vi "Robot Global Data.vi"() -> ()   [LabVIEW 2017]
doc: "This global VI can contain as many global variables as you need. Place a control on the panel, give it a good name. To read or write to it from a VI, drag the icon to the diagram of that VI. You can also drag from the project. Click on the node to change which global you access. You shouldn't have multiple locations writing to a global or it will cause a race-condition."
uses:
  <vilib>/Rock Robotics/WPI/Camera/WPI_CameraImageSize.ctl
  <vilib>/Rock Robotics/WPI/DriverStation/WPI_DriverStationRobotMode2.ctl
  Common Code/Dashboard Control Data.ctl
  Common Code/Drivetrain Command Cluster.ctl
  Common Code/Drivetrain Mode.ctl
  Common Code/Drivetrain Status Cluster.ctl
  Common Code/Climb Command Cluster.ctl
  Common Code/Climb Status Cluster.ctl
  Common Code/DT Encoder Values.ctl
panel:
  in  "Drivetrain Encoder Values":T1
  in  "Climb Status Cluster":T2
  in  "Climb Command Cluster":T3
  out "Drivetrain Status Cluster":T4 {"Gyro" scale=-180.0..180.0}
  in  "Drivetrain Command Cluster":T6
  in  "Dashboard Control Data":T7
  in  "Driver Station IP":dbl
  in  "Robot Mode":T8
  in  "image size":T9=enum."320x240"
  in  "Enable Vision":bool
  # "Dashboard"
  # "Drivetrain"
  # "Intake"
  # "Climber"
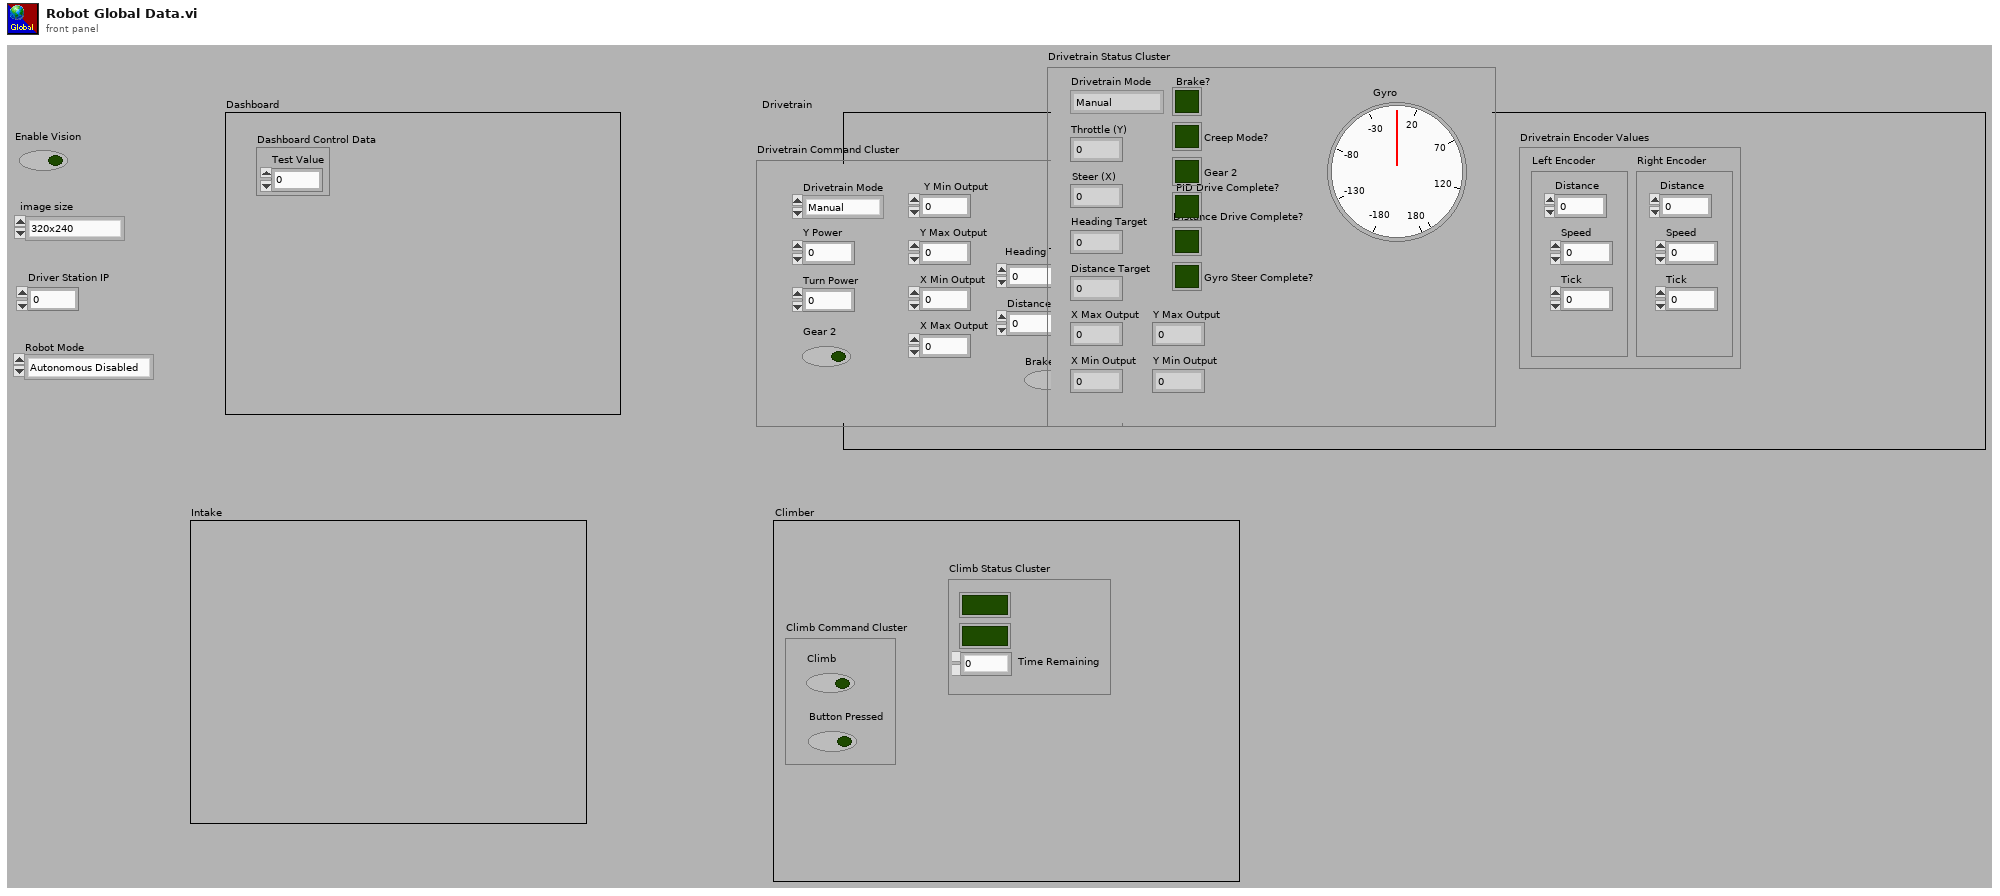
[diagram p1: front panel]
types:
  T1 = typedef "DT Encoder Values.ctl" = cluster{"Left Encoder":cluster{"Distance":dbl, "Speed":dbl, "Tick":dbl}, "Right Encoder":cluster{"Distance":dbl, "Speed":dbl, "Tick":dbl}}
  T2 = typedef "Climb Status Cluster.ctl" = cluster{"Climb":bool, "Button Pressed":bool, "Time Remaining":dbl}
  T3 = typedef "Climb Command Cluster.ctl" = cluster{"Climb":bool, "Button Pressed":bool}
  T4 = typedef "Drivetrain Status Cluster.ctl" = cluster{"Throttle (Y)":dbl, "Steer (X)":dbl, "Drivetrain Mode":T5, "Brake?":bool, "Distance Drive Complete?":bool, "PID Drive Complete?":bool, "Creep Mode?":bool, "Gyro Steer Complete?":bool, "Gyro":dbl, "X Max Output":dbl, "X Min Output":dbl, "Y Max Output ":dbl, "Y Min Output":dbl, "Heading Target":dbl, "Distance Target":dbl, "Gear 2":bool}
  T5 = typedef "Drivetrain Mode.ctl" = enum16{"Manual", "Gyro Steer", "PID Drive", "Distance Drive", "Autonomous"}
  T6 = typedef "Drivetrain Command Cluster.ctl" = cluster{"Y Power":dbl, "Turn Power":dbl, "Drivetrain Mode":T5, "Gear 2":bool, "Y Min Output":dbl, "Y Max Output":dbl, "X Min Output":dbl, "X Max Output":dbl, "Heading Target":dbl, "Distance Target":dbl, "Brake?":bool}
  T7 = typedef "Dashboard Control Data.ctl" = cluster{"Test Value":dbl}
  T8 = typedef "WPI_DriverStationRobotMode2.ctl" = enum16{"Autonomous Disabled", "Autonomous Enabled", "Teleop Disabled", "Teleop Enabled", "Disconnected", "Finish", "Test Disabled", "Test Enabled", "Emergency Stopped"}
  T9 = typedef "WPI_CameraImageSize.ctl" = enum16{"640x480", "320x240", "160x120", "Custom"}
diagram:
